vi "2.4.-GUI Filtros RGB.vi"() -> ()   [LabVIEW 2020]
panel:
  in  "Enum":T1(ring)
  in  "Path":path
  in  "U3 gris":u8(slide) scale=0.0..255.0
  in  "U2 gris":u8(slide) scale=0.0..255.0
  in  "U1 gris":u8(slide) scale=0.0..255.0
  out "q = Img Filtro":picture
  in  "U inf":u8(slide) scale=0.0..255.0
  in  "U sup":u8(slide) scale=0.0..255.0
  out "p = Img Original":picture
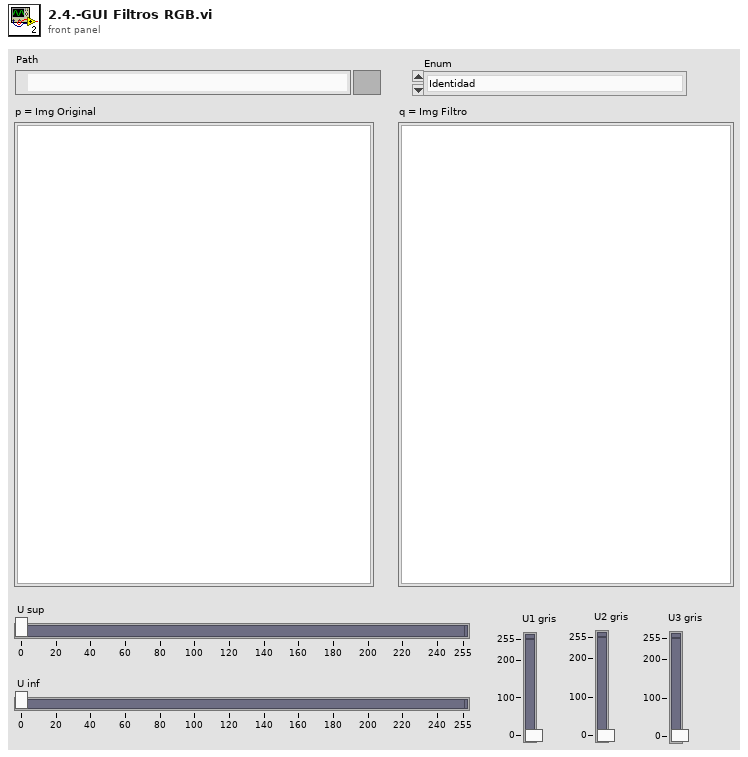
[diagram p1: front panel]
types:
  T1 = enum8{"Identidad", "Inverso", "Umbral", "Umbral Binario", "Umbral Binario Invertido", "Umbral Escala Grises", "Umbral Escala Grises Inv", "Extensión", "Reducción Nivel Grises", ""}
  T2 = typedef "imagedata.ctl" = cluster{"image type":i32, "image depth":i32, "image":u8[], "mask":u8[], "colors":u32[], "Rectangle":cluster{"left":i16, "top":i16, "right":i16, "bottom":i16}}
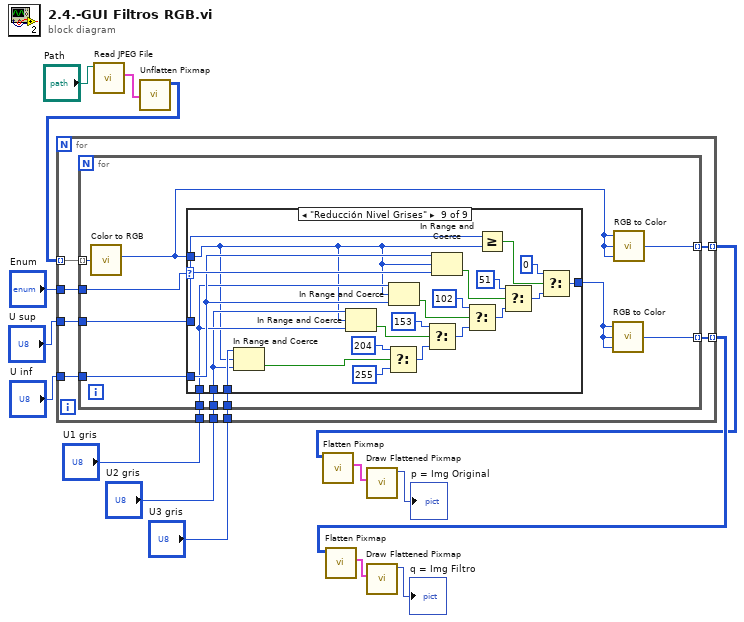
[diagram p0: block diagram]
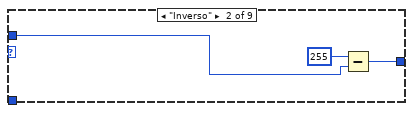
[diagram p3: hidden frame]
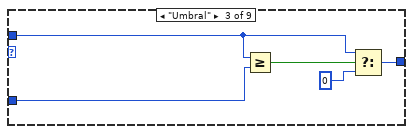
[diagram p4: hidden frame]
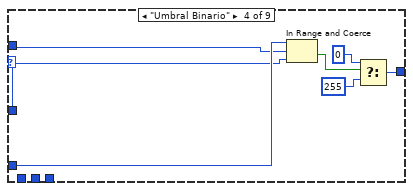
[diagram p5: hidden frame]
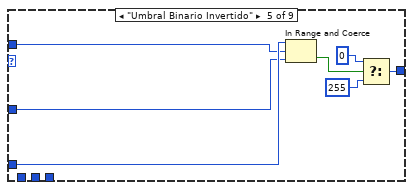
[diagram p6: hidden frame]
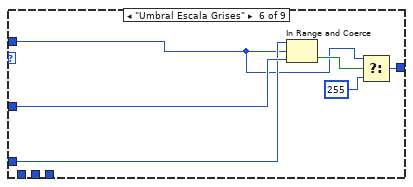
[diagram p7: hidden frame]
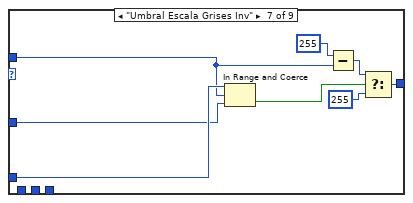
[diagram p8: hidden frame]
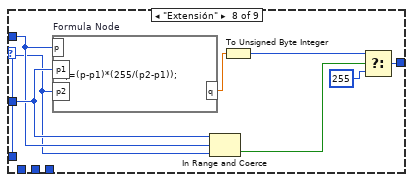
[diagram p9: hidden frame]
diagram:
  n1 = call <vilib>:"Read JPEG File.vi"("path to JPEG file"="Path") -> ("image data"=w14:T2)  [unwired: 8 in, 2 out]
  n2 = call <vilib>:"Unflatten Pixmap.vi"("image data"=w14) -> ("24-bit pixmap"=w13:u32[][])  [unwired: 4 in, 6 out]
  n3 = for {
    tunnel: w13 -> [w24] mode=indexing
    tunnel: "U sup" -> [w23]
    tunnel: "U inf" -> [w22]
    tunnel: [w21] -> w10 mode=indexing
    tunnel: "U1 gris" -> [w20]
    tunnel: "U2 gris" -> [w19]
    tunnel: "U3 gris" -> [w18]
    tunnel: "Enum" -> [w17]
    tunnel: [w16] -> w3 mode=indexing
    n4 = for {
      tunnel: w24 -> [w35] mode=indexing
      tunnel: w23 -> [w34]
      tunnel: w22 -> [w33]
      tunnel: [w31] -> w21 mode=indexing
      tunnel: w20 -> [w30]
      tunnel: w19 -> [w29]
      tunnel: w18 -> [w28]
      tunnel: w17 -> [w27]
      tunnel: [w26] -> w16 mode=indexing
      n5 = call <vilib>:"Color to RGB.vi"("Color"=w35) -> ("R"=w25:u8)  [unwired: 3 out]
      n6 = case shown="\"Reducción Nivel Grises\"" w27 {
        tunnel: w25 -> [w36 w38 w42 w48 w53 w60 w67 w75 w81]
        tunnel: w34 -> [_ _ w41 w47 w54 w62 w69 w76 w86]
        tunnel: w33 -> [_ _ _ w49 w55 w61 w70 w74 w85]
        tunnel: [w36 w37 w40 w45 w52 w59 w65 w73 w87] -> w32
        tunnel: w30 -> [_ _ _ _ _ _ _ _ w84]
        tunnel: w29 -> [_ _ _ _ _ _ _ _ w82]
        tunnel: w28 -> [_ _ _ _ _ _ _ _ w83]
        frame "Identidad", Default {
        }
        frame "Inverso" {
          n7 = Subtract(x=255, y=w38) -> (x-y=w37:i32)
        }
        frame "Umbral" {
          n8 = Greater Or Equal?(x=w42, y=w41) -> (x >= y?=w44:bool)
          n9 = Select(t=w42, s=w44, f=u8 0) -> (s? t:f=w40:u8)
        }
        frame "Umbral Binario" {
          n10 = In Range and Coerce(upper limit=w49, x=w48, lower limit=w47) -> (In Range?=w46:bool)  [unwired: 1 out]
          n11 = Select(t=0, s=w46, f=255) -> (s? t:f=w45:i32)
        }
        frame "Umbral Binario Invertido" {
          n12 = In Range and Coerce(upper limit=w55, x=w53, lower limit=w54) -> (In Range?=w56:bool)  [unwired: 1 out]
          n13 = Select(t=0, s=w56, f=255) -> (s? t:f=w52:i32)
        }
        frame "Umbral Escala Grises" {
          n14 = In Range and Coerce(upper limit=w61, x=w60, lower limit=w62) -> (In Range?=w63:bool)  [unwired: 1 out]
          n15 = Select(t=w60, s=w63, f=255) -> (s? t:f=w59:i32)
        }
        frame "Umbral Escala Grises Inv" {
          n16 = In Range and Coerce(upper limit=w70, x=w67, lower limit=w69) -> (In Range?=w71:bool)  [unwired: 1 out]
          n17 = Subtract(x=255, y=w67) -> (x-y=w66:i32)
          n18 = Select(t=w66, s=w71, f=255) -> (s? t:f=w65:i32)
        }
        frame "Extensión" {
          n19 = formula code="q=(p-p1)*(255/(p2-p1));"("p"=w75, "p1"=w76, "p2"=w74) -> ("q"=w80:dbl)
          n20 = In Range and Coerce(upper limit=w76, x=w75, lower limit=w74) -> (In Range?=w79:bool)  [unwired: 1 out]
          n21 = To Unsigned Byte Integer(number=w80) -> (unsigned 8bit integer=w77:u8)
          n22 = Select(t=w77, s=w79, f=255) -> (s? t:f=w73:i32)
        }
        frame "Reducción Nivel Grises" {
          n23 = In Range and Coerce(upper limit=w83, x=w81, lower limit=w82) -> (In Range?=w91:bool)  [unwired: 1 out]
          n24 = In Range and Coerce(upper limit=w82, x=w81, lower limit=w84) -> (In Range?=w92:bool)  [unwired: 1 out]
          n25 = Select(t=u8 204, s=w91, f=u8 255 ("t")) -> (s? t:f=w89:u8)
          n26 = In Range and Coerce(upper limit=w84, x=w81, lower limit=w85) -> (In Range?=w96:bool)  [unwired: 1 out]
          n27 = Select(t=u8 153, s=w92, f=w89) -> (s? t:f=w93:u8)
          n28 = In Range and Coerce(upper limit=w85, x=w81, lower limit=w86) -> (In Range?=w100:bool)  [unwired: 1 out]
          n29 = Select(t=u8 102, s=w96, f=w93) -> (s? t:f=w97:u8)
          n30 = Greater Or Equal?(x=w86, y=w81) -> (x >= y?=w102:bool)
          n31 = Select(t=u8 51, s=w100, f=w97) -> (s? t:f=w98:u8)
          n32 = Select(t=0, s=w102, f=w98) -> (s? t:f=w87:i32)
        }
      }
      n33 = call <vilib>:"RGB to Color.vi"("B"=w32, "G"=w32, "R"=w32) -> ("Color"=w31:u32)
      n34 = call <vilib>:"RGB to Color.vi"("B"=w25, "G"=w25, "R"=w25) -> ("Color"=w26:u32)
    }
  }
  n35 = call <vilib>:"Flatten Pixmap.vi"("24-bit pixmap"=w3) -> ("image data"=w4:T2)  [unwired: 10 in]
  n36 = call <vilib>:"Flatten Pixmap.vi"("24-bit pixmap"=w10) -> ("image data"=w9:T2)  [unwired: 10 in]
  n37 = call <vilib>:"Draw Flattened Pixmap.vi"("image data"=w4) -> ("new picture"=→"p = Img Original":picture)  [unwired: 8 in]
  n38 = call <vilib>:"Draw Flattened Pixmap.vi"("image data"=w9) -> ("new picture"=→"q = Img Filtro":picture)  [unwired: 8 in]
